vi "CreateColor.vi"(8 "error in (no error)":errorcluster, 9 "ColorsIn":T1(c390), 10 "Color(Black)":u32, 11 "Alpha(100%)":dbl=100.0) -> (0 "error out":errorcluster, 1 "ColorsOut":T1(c390), 3 "ColorRef":refnum<k24>)   [LabVIEW 2020, in "LcPictureBox.lvclass"]
uses:
  LcPictureBox.lvclass
  System.Drawing
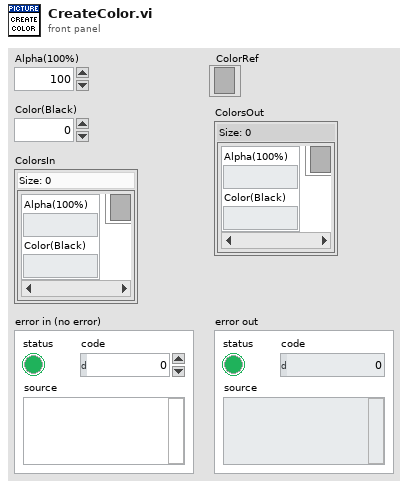
[diagram p1: front panel]
types:
  T1 = map{cluster{"Alpha(100%)":dbl, "Color(Black)":u32}, refnum<k24>}
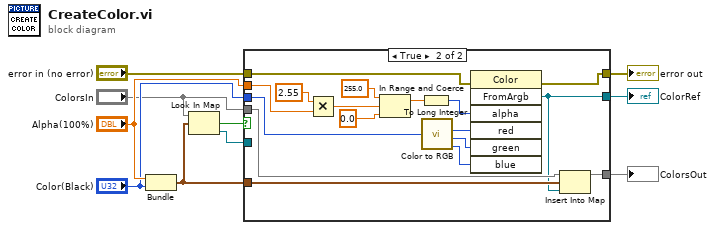
[diagram p0: block diagram]
diagram:
  n1 = Bundle("Alpha(100%)"="Alpha(100%)", "Color(Black)"="Color(Black)") -> (w1:cluster{"Alpha(100%)":dbl, "Color(Black)":u32})  [unwired: 1 in]
  n2 = Look In Map(map="ColorsIn", key=w1) -> (key not found?=w4:bool, value=w5:refnum<k24>)  [unwired: 1 in]
  n3 = case shown="True" w4 {
    tunnel: [w13 w14] -> w10
    tunnel: "Alpha(100%)" -> [_ w21]
    tunnel: "Color(Black)" -> [_ w20]
    tunnel: "error in (no error)" -> [w12 w19]
    tunnel: [w12 w18] -> w6
    tunnel: w5 -> [w13 _]
    tunnel: "ColorsIn" -> [w11 w17]
    tunnel: [w11 w16] -> w2
    tunnel: w1 -> [_ w15]
    frame False {
    }
    frame True {
      n4 = Multiply(x=2.55, y=w21) -> (x*y=w27:dbl)
      n5 = In Range and Coerce(upper limit=255.0, x=w27, lower limit=0.0) -> (coerced(x)=w30:dbl)  [unwired: 1 out]
      n6 = To Long Integer(number=w30) -> (32bit integer=w22:i32)
      n7 = call <vilib>:"Color to RGB.vi"("Color"=w20) -> ("R"=w23:u8, "G"=w24:u8, "B"=w25:u8)  [unwired: 1 out]
      n8 = invoke class="Color" method="FromArgb"(error in=w19, "alpha"=w22, "red"=w23, "green"=w24, "blue"=w25) -> (error out=w18:errorcluster, "FromArgb"=w14:refnum<k24>)  [unwired: 2 in, 5 out]
      n9 = Insert Into Map(map in=w17, key=w15, value=w14) -> (map out=w16:T1)  [unwired: 2 out]
    }
  }
  "ColorRef" <- w10
  "error out" <- w6
  "ColorsOut" <- w2
